vi "MANUAL_COMMAND_SCREEN.vi"() -> ()   [LabVIEW 2017]
panel:
  out "Boolean Rectangle 8":bool
  out "Boolean Rectangle 7":bool
  out "Boolean Rectangle 6":bool
  out "Boolean Rectangle 5":bool
  out "Boolean Rectangle 4":bool
  out "Boolean Rectangle 3":bool
  out "Boolean Rectangle 2":bool
  out "Boolean Rectangle":bool
  in  "Down 2":bool
  in  "Up 2":bool
  in  "Add Button":bool
  in  "RIGHT":bool
  in  "LEFT":bool
  in  "Down":bool
  in  "Up":bool
  in  "Close":bool
  # "RBC ORVM- MANUAL COMMAND SCREEN"
  # "PFLOD"
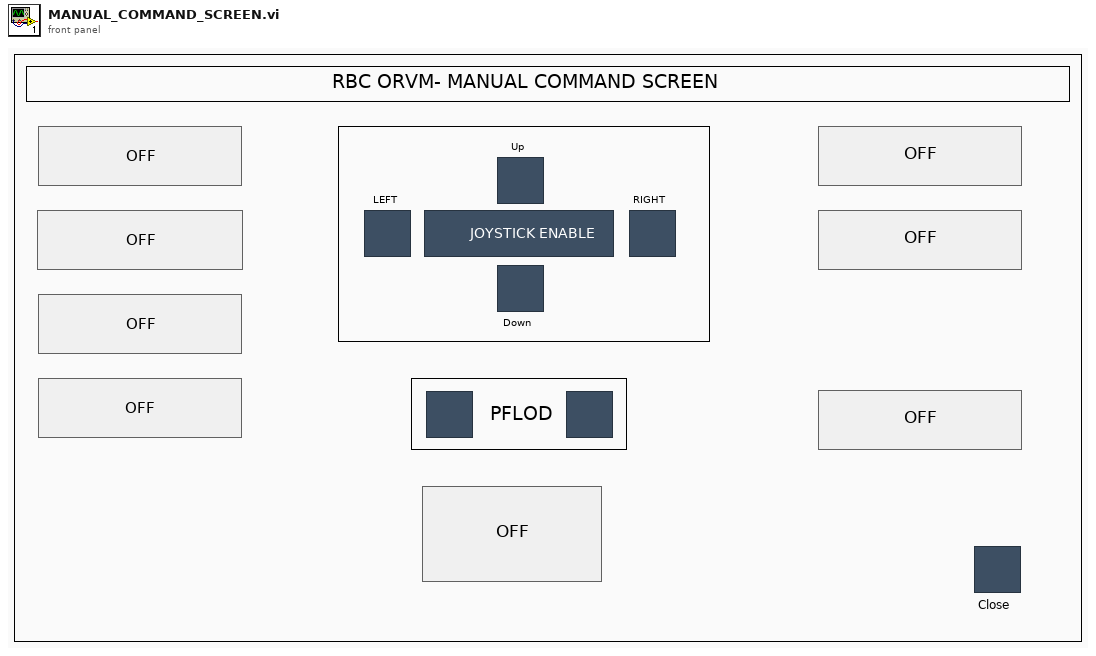
[diagram p1: front panel]
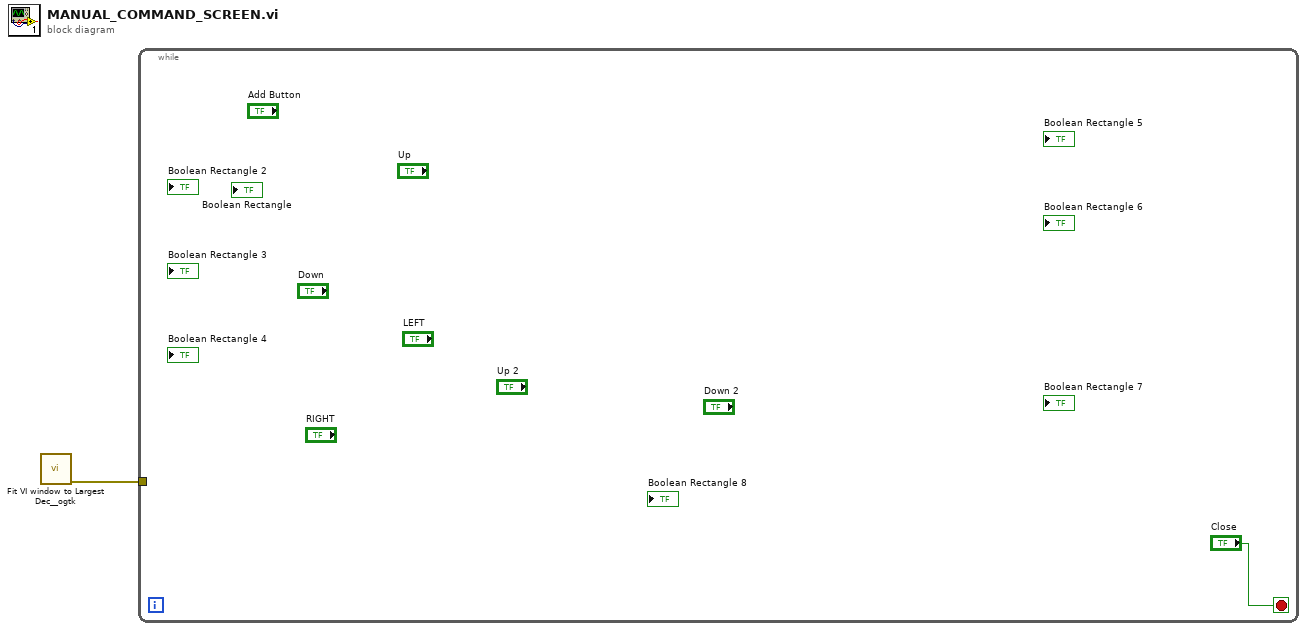
[diagram p0: block diagram]
diagram:
  n1 = call <userlib>:"Fit VI window to Largest Dec__ogtk.vi"() -> ("error out"=w1:errorcluster)  [unwired: 6 in, 1 out]
  n2 = while {
    tunnel: w1 -> [_]
    stop <- "Close" stop-if-true
  }
